vi "encode_test_HOST.vi"() -> ()   [LabVIEW 2014]
uses:
  <vilib>/userdefined/High Color/nirio_resource_hc.ctl
  <vilib>/addons/h5labview2/file/H5Fmode.ctl
  <vilib>/FPGAPlugInAG/PXI-7854R/niLvFpga_Open_PXI-7854R.vi
  <vilib>/rvi/interface/common/dynamic/niFpgaDynamicAddResources.vi
  <vilib>/FPGAPlugInAG/Dynamic/niLvFpga_Run_Dynamic.vi
  <vilib>/Utility/error.llb/Error Cluster From Error Code.vi
  <vilib>/rvi/errors/niLvFpgaAdjustHostInterfaceError.vi
  <vilib>/addons/h5labview2/base/lib_path.vi
  <vilib>/addons/h5labview2/base/H5Equery.vi
  <vilib>/FPGAPlugInAG/Dynamic/niLvFpga_Close_Dynamic.vi
  <vilib>/rvi/interface/nirviOpenFPGA/nirviOpenFPGA.xnode
  FPGA Bitfiles/encodetest,lvpro_FPGATarget_encodetestFPGA_g0rLf42jriM.lvbitx
  <vilib>/rvi/interface/nirviMethod/nirviMethod.xnode
  <vilib>/rvi/interface/nirviReadWriteControl/nirviReadWriteControl.xnode
  <vilib>/addons/h5labview2/base/hid_t.ctl
  <vilib>/addons/h5labview2/dataset/H5Dwrite.llb/H5Dwrite.xnode
  <vilib>/rvi/interface/nirviCloseFPGA/nirviCloseFPGA.xnode
  NiFpgaLv.dll
  <vilib>/rvi/interface/Simulation/niFpgaSimulationCallBeginRW.vi
  <vilib>/rvi/errors/niLvFpgaMergeErrorWithErrorCode.vi
  <vilib>/FPGAPlugInAG/Dynamic/niLvFpga_ReadFifo_Dynamic.vi
  <vilib>/addons/h5labview2/file/H5F.lvlib
  <vilib>/addons/h5labview2/group/H5G.lvlib
  <vilib>/FPGAPlugInAG/Dynamic/niLvFpga_StartFifo_Dynamic.vi
  <vilib>/FPGAPlugInAG/Dynamic/niLvFpga_StopFifo_Dynamic.vi
panel:
  out "loop time":fxp<+,32,32>
  in  "wait (usec)":u32
  in  "Host Update Rate (msec)":dbl=1.0 format="%#_13g"
  in  "Update ADC Clock":bool
  in  "loop timer (usec)":u32=2
  in  "accept_trigs":bool=TRUE
  in  "reset_trigs":bool
  out "config_loaded":bool
  out "fpga_dat_path":path=path "C:/Data/20180605/bead1/discharge/coarse2/turbombar_xyzcool_lessfb_elec3_3000mV41Hz0mVdc_25_fpga.h5"
  out "Nsamp_config":u32=50000
  out "config_trig":bool
  in  "block_hardware_trigs":bool
  out "TRIG0":bool=TRUE
  out "TRIG1":bool=TRUE
  in  "RIO Device":T1="RIO0"
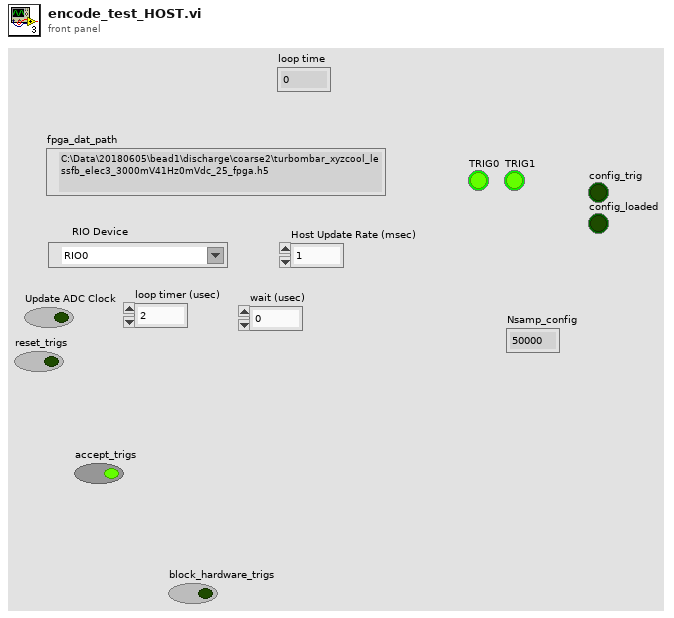
[diagram p1: front panel]
types:
  T1 = typedef "nirio_resource_hc.ctl" = tag
  T2 = enum16{"open", "replace", "create", "open or create", "replace or create", "replace or create with confirmation"}
  T3 = typedef "H5F.lvlib/H5Fmode.ctl" = enum16{"read-only", "read-write", "overwrite", "create new", "open or create"}
  T4 = typedef "hid_t.ctl" = i32
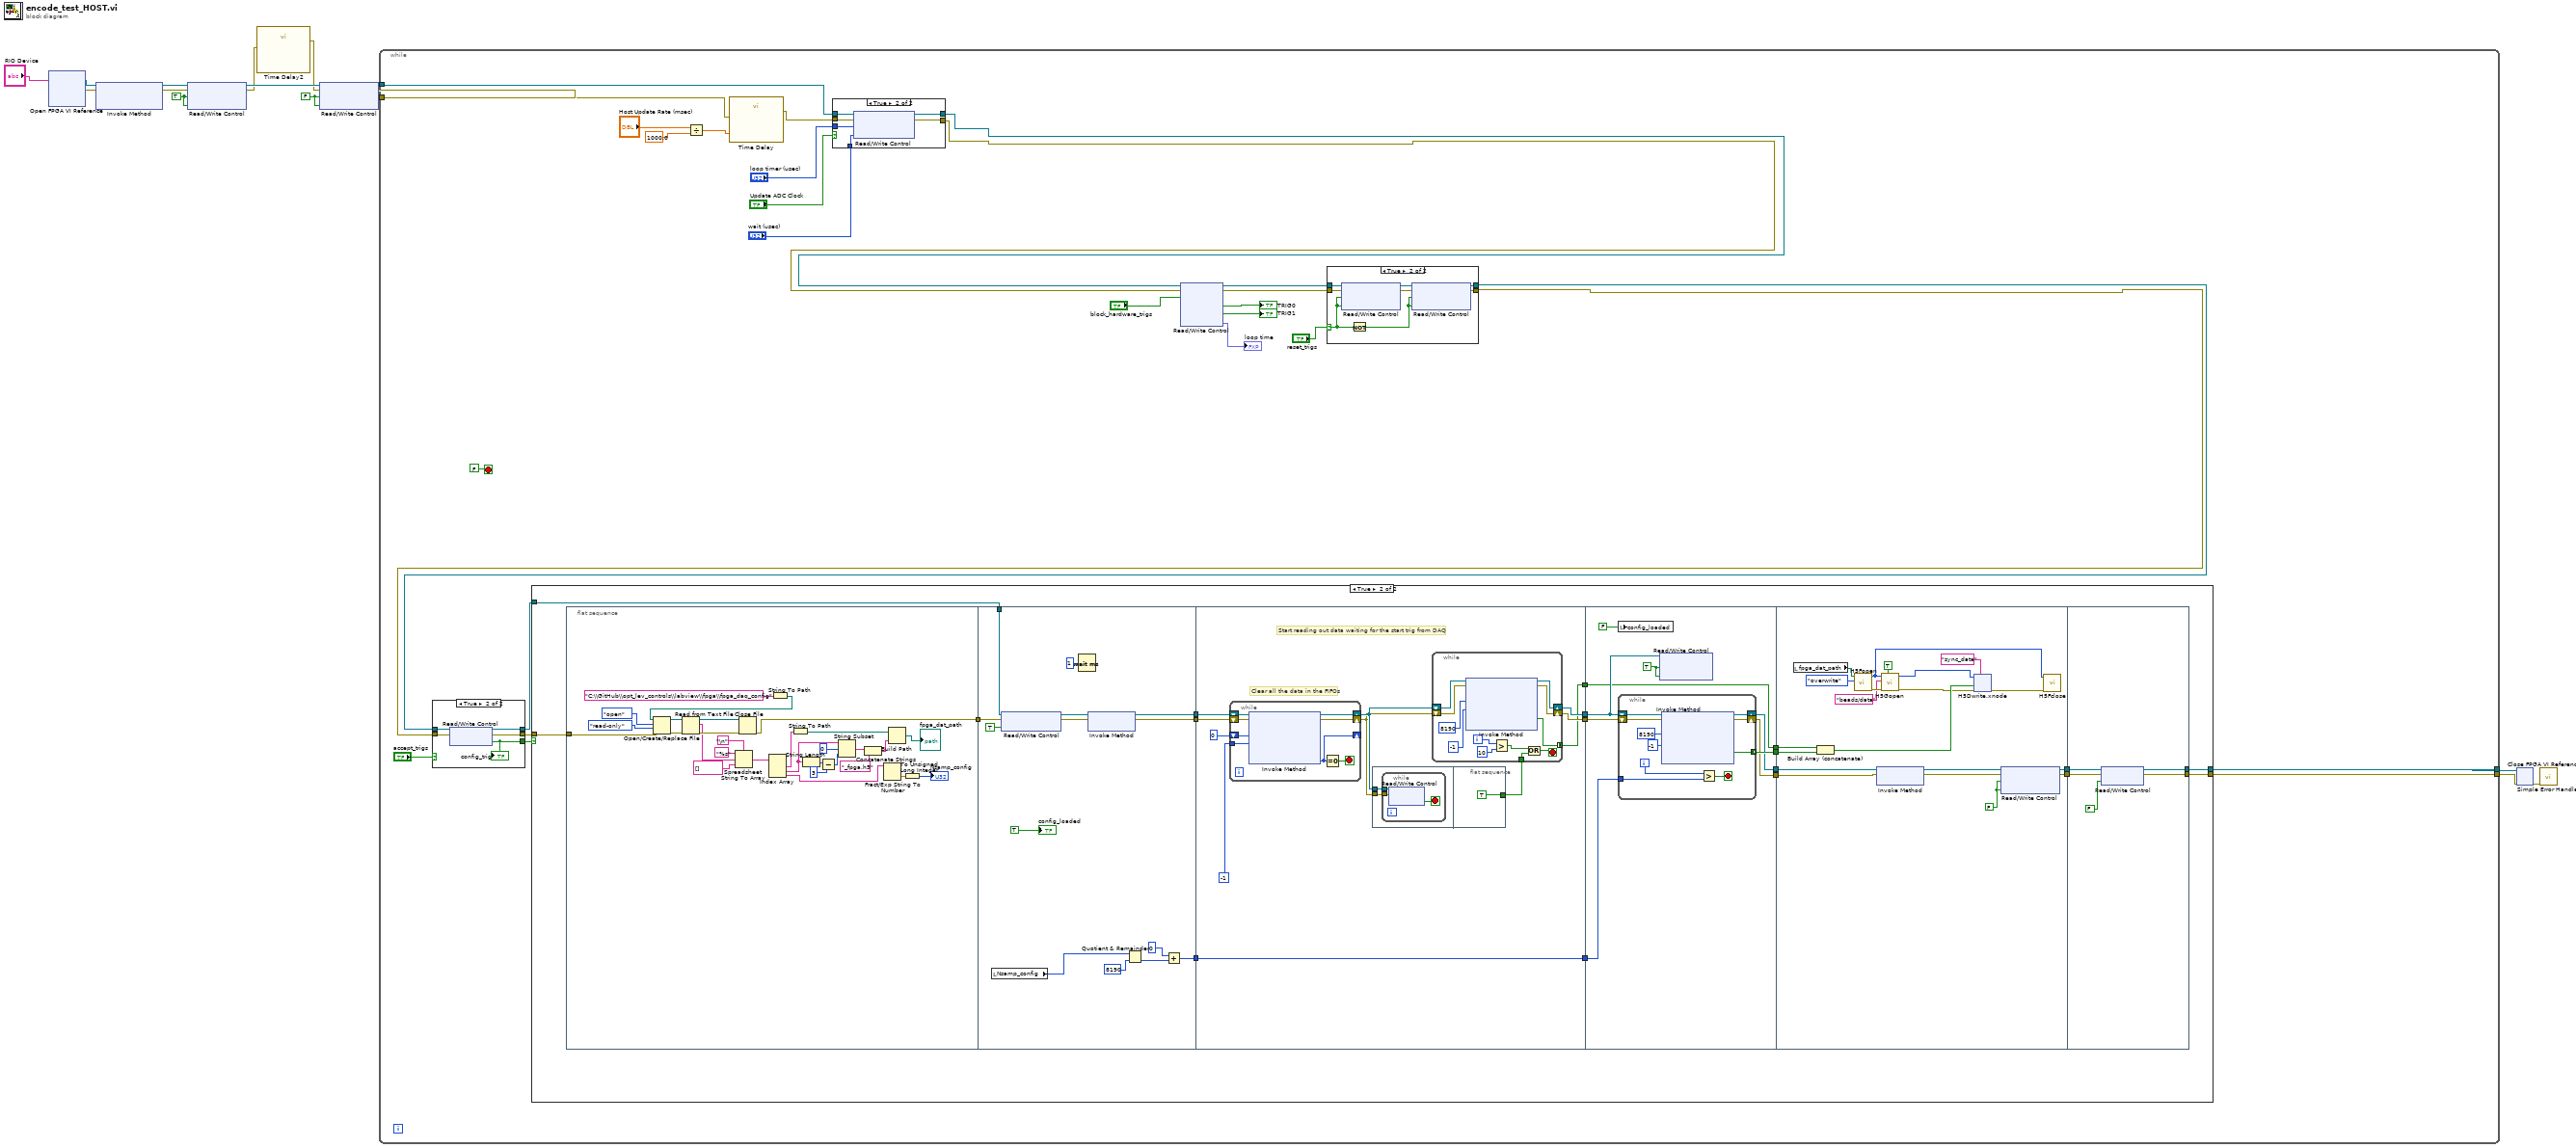
[diagram p0: block diagram]
diagram:
  w5 = FALSE ("manual_trig")
  w3 = TRUE ("reset_trig")
  n1 = xnode "Open FPGA VI Reference"("resource name"="RIO Device") -> ("FPGA VI Reference Out"=w11:refnum<k20>, "error out"=w10:errorcluster)  [unwired: 1 in]
  n2 = xnode "Invoke Method"("FPGA VI Reference In"=w11, "error in"=w10) -> ("FPGA VI Reference Out"=w9:refnum<k20>, "error out"=w8:errorcluster)  [unwired: 1 in]
  n3 = xnode "Read/Write Control"("FPGA VI Reference In"=w9, "error in"=w8, "reset_data_trig"=w3, "reset_config_trig"=w3) -> ("FPGA VI Reference Out"=w4:refnum<k20>, "error out"=w2:errorcluster)
  n4 = call "Time Delay2"("error in (no error)"=w2) -> ("error out"=w1:errorcluster)  [unwired: 10 in]
  n5 = xnode "Read/Write Control"("FPGA VI Reference In"=w4, "error in"=w1, "reset_data_trig"=w5, "reset_config_trig"=w5) -> ("FPGA VI Reference Out"=w7:refnum<k20>, "error out"=w6:errorcluster)
  n6 = while {
    tunnel: w6 -> [w41]
    tunnel: w7 -> [w39]
    tunnel: [w23] -> w14
    tunnel: [w22] -> w13
    stop <- FALSE stop-if-true
    n7 = Divide(x="Host Update Rate (msec)", y=1000.0) -> (x/y=w42:dbl)
    n8 = call "Time Delay"("error in (no error)"=w41, "Delay Time (s)"=w42) -> ("error out"=w38:errorcluster)  [unwired: 9 in]
    n9 = case shown="True" "Update ADC Clock" {
      tunnel: w39 -> [w224 w230]
      tunnel: w38 -> [w223 w229]
      tunnel: [w224 w228] -> w19
      tunnel: [w223 w227] -> w18
      tunnel: "loop timer (usec)" -> [_ w226]
      tunnel: "wait (usec)" -> [_ w225]
      frame False {
      }
      frame True {
        n10 = xnode "Read/Write Control"("FPGA VI Reference In"=w230, "error in"=w229, "loop timer (usec)"=w226, "wait (usec)"=w225) -> ("FPGA VI Reference Out"=w228:refnum<k20>, "error out"=w227:errorcluster)
      }
    }
    n11 = xnode "Read/Write Control"("FPGA VI Reference In"=w19, "error in"=w18, "block_trigs"="block_hardware_trigs") -> ("FPGA VI Reference Out"=w33:refnum<k20>, "error out"=w32:errorcluster, "TRIG0"=→"TRIG0":bool, "TRIG1"=→"TRIG1":bool, "loop time"=→"loop time":fxp<+,32,32>)
    n12 = case shown="True" "reset_trigs" {
      selector: "reset_trigs" -> [_ w216]
      tunnel: w33 -> [w214 w222]
      tunnel: w32 -> [w213 w221]
      tunnel: [w214 w218] -> w21
      tunnel: [w213 w217] -> w20
      frame False {
      }
      frame True {
        n13 = xnode "Read/Write Control"("FPGA VI Reference In"=w222, "error in"=w221, "reset_data_trig"=w216, "reset_config_trig"=w216) -> ("FPGA VI Reference Out"=w220:refnum<k20>, "error out"=w219:errorcluster)
        n14 = Not(x=w216) -> (.not. x?=w215:bool)
        n15 = xnode "Read/Write Control"("FPGA VI Reference In"=w220, "error in"=w219, "reset_data_trig"=w215, "reset_config_trig"=w215) -> ("FPGA VI Reference Out"=w218:refnum<k20>, "error out"=w217:errorcluster)
      }
    }
    n16 = case shown="True" "accept_trigs" {
      selector: "accept_trigs" -> [w45 _]
      tunnel: [w45 w50] -> w29
      tunnel: w20 -> [w43 w49]
      tunnel: w21 -> [w44 w48]
      tunnel: [w44 w47] -> w28
      tunnel: [w43 w46] -> w27
      frame False {
      }
      frame True {
        n17 = xnode "Read/Write Control"("FPGA VI Reference In"=w48, "error in"=w49) -> ("FPGA VI Reference Out"=w47:refnum<k20>, "error out"=w46:errorcluster, "config_trig"=w50:bool)
        "config_trig" <- w50
      }
    }
    n18 = case shown="True" w29 {
      tunnel: w28 -> [w52 w69]
      tunnel: [w52 w58] -> w23
      tunnel: [w51 w57] -> w22
      tunnel: w27 -> [w51 w54]
      frame False {
      }
      frame True {
        n19 = flat-sequence {
          tunnel: [w91] -> w70
          tunnel: w54 -> [w71]
          tunnel: w70 -> [w105]
          tunnel: w69 -> [w106]
          tunnel: [w103] -> w68
          tunnel: [w104] -> w64
          tunnel: [w100] -> w53
          tunnel: w68 -> [w116]
          tunnel: [w120] -> w67
          tunnel: [w119] -> w66
          tunnel: [w118] -> w65
          tunnel: w64 -> [w118]
          tunnel: [w117] -> w62
          tunnel: w53 -> [w115]
          tunnel: w67 -> [w157]
          tunnel: w66 -> [w159]
          tunnel: w65 -> [w158]
          tunnel: [w156] -> w63
          tunnel: w62 -> [w156]
          tunnel: [w155] -> w61
          tunnel: [w154] -> w60
          tunnel: [w153] -> w59
          tunnel: w63 -> [w179]
          tunnel: w61 -> [w178]
          tunnel: w60 -> [w176]
          tunnel: w59 -> [w175]
          tunnel: [w174] -> w56
          tunnel: [w173] -> w55
          tunnel: [w208] -> w57
          tunnel: [w209] -> w58
          tunnel: w56 -> [w211]
          tunnel: w55 -> [w210]
          frame #0 {
            n20 = String To Path(string="C:\\GitHub\\opt_lev_controls\\labview\\fpga\\fpga_daq_config") -> (path=w98:path)
            n21 = Open/Create/Replace File(file path (use dialog)=w98, error in=w71, operation (0:open)=T2."open", access (0:read/write)=enum16{"read/write", "read-only", "write-only"}."read-only") -> (refnum out=w95:refnum<file>, error out=w94:errorcluster)  [unwired: 2 in, 1 out]
            n22 = Read from Text File(file (use dialog)=w95, error in=w94) -> (refnum out=w93:refnum<file>, text=w90:string, error out=w92:errorcluster)  [unwired: 2 in, 1 out]
            n23 = Spreadsheet String To Array(delimiter (Tab)="\n", format string="%s", spreadsheet string=w90, array type (2D Dbl)=string[] [] ("array of strings")) -> (array=w86:string[])
            n24 = Close File(refnum=w93, error in=w92) -> (error out=w91:errorcluster)  [unwired: 1 out]
            n25 = Index Array(array=w86) -> (element #1=w85:string, element #2=w82:string, element #3=w74:string)  [unwired: 3 in]
            n26 = String To Path(string=w85) -> (path=w84:path)
            n27 = String Length(string=w82) -> (length=w81:i32)
            n28 = Subtract(x=w81, y=3) -> (x-y=w79:i32)
            n29 = String Subset(string=w82, offset (0)=0, length (rest)=w79) -> (substring=w78:string)
            n30 = Concatenate Strings(w78, "_fpga.h5" ("string")) -> (w76:string)
            n31 = Fract/Exp String To Number(string=w74) -> (number=w73:dbl)  [unwired: 3 in, 1 out]
            n32 = Build Path(base path=w84, name or relative path=w76) -> (appended path=→"fpga_dat_path":path)
            n33 = To Unsigned Long Integer(number=w73) -> (unsigned 32bit integer=→"Nsamp_config":u32)
          }
          frame #1 {
            n34 = local read "Nsamp_config"() -> (w101:u32)
            n35 = xnode "Read/Write Control"("FPGA VI Reference In"=w106, "error in"=w105, "reset_config_trig"=TRUE) -> ("FPGA VI Reference Out"=w107:refnum<k20>, "error out"=w108:errorcluster)
            n36 = Wait (ms)(milliseconds to wait=u32 1) -> ()  [unwired: 1 out]
            n37 = xnode "Invoke Method"("FPGA VI Reference In"=w107, "error in"=w108) -> ("FPGA VI Reference Out"=w103:refnum<k20>, "error out"=w100:errorcluster)
            n38 = Quotient & Remainder(x=w101, y=u32 8190) -> (floor(x/y)=w111:u32)  [unwired: 1 out]
            n39 = Add(x=u32 0 ("Extra Samps"), y=w111) -> (x+y=w104:u32)
            "config_loaded" <- TRUE
          }
          frame #2 {
            # "Start reading out data waiting for the start trig from DAQ"
            # "Clear all the data in the FIFOs"
            n40 = while {
              tunnel: -1 -> [w145]
              shift-right: [w147] -> w122
              shift-left: w116 -> [w150]
              shift-right: [w146] -> w121
              shift-left: w115 -> [w149]
              shift-right: [w144] -> _
              shift-left: u32 0 ("Elements Remaining") -> [w148]
              stop <- w143 stop-if-true
              n41 = xnode "Invoke Method"("FPGA VI Reference In"=w150, "error in"=w149, "Number of Elements"=w148, "Timeout (ms)"=w145) -> ("FPGA VI Reference Out"=w147:refnum<k20>, "error out"=w146:errorcluster, "Elements Remaining"=w144:u32)  [unwired: 1 out]
              n42 = Equal To 0?(x=w144) -> (x = 0?=w143:bool)
            }
            n43 = flat-sequence {
              tunnel: w122 -> [w126]
              tunnel: w121 -> [w125]
              tunnel: [TRUE] -> w114
              frame #0 {
                n44 = while {
                  tunnel: w126 -> [w129]
                  tunnel: w125 -> [w128]
                  stop <- w127 stop-if-true
                  n45 = xnode "Read/Write Control"("FPGA VI Reference In"=w129, "error in"=w128) -> ("data_trig"=w127:bool)  [unwired: 2 out]
                }
              }
              frame #1 {
              }
            }
            n46 = while {
              tunnel: [w138] -> w117 mode=concatenating
              shift-right: [w140] -> w120
              shift-left: w122 -> [w142]
              shift-right: [w139] -> w119
              shift-left: w121 -> [w141]
              tunnel: w114 -> [w133]
              i -> [w136]
              stop <- w132 stop-if-true
              n47 = xnode "Invoke Method"("FPGA VI Reference In"=w142, "error in"=w141, "Number of Elements"=u32 8190, "Timeout (ms)"=-1) -> ("FPGA VI Reference Out"=w140:refnum<k20>, "error out"=w139:errorcluster, "Data"=w138:bool[])  [unwired: 1 out]
              n48 = Greater?(x=w136, y=10) -> (0:w134:bool)
              n49 = Or(x=w134, y=w133) -> (x .or. y?=w132:bool)
            }
          }
          frame #3 {
            w152 = TRUE
            n50 = local write "config_loaded"(FALSE) -> ()
            n51 = while {
              shift-right: [w165] -> w154
              shift-left: w157 -> [w169]
              shift-right: [w164] -> w153
              shift-left: w159 -> [w168]
              tunnel: w158 -> [w161]
              tunnel: [w160] -> w155 mode=concatenating
              i -> [w163]
              stop <- w162 stop-if-true
              n52 = xnode "Invoke Method"("FPGA VI Reference In"=w169, "error in"=w168, "Number of Elements"=u32 8190, "Timeout (ms)"=-1) -> ("FPGA VI Reference Out"=w165:refnum<k20>, "error out"=w164:errorcluster, "Data"=w160:bool[])  [unwired: 1 out]
              n53 = Greater?(x=w163, y=w161) -> (0:w162:bool)
            }
            n54 = xnode "Read/Write Control"("FPGA VI Reference In"=w157, "reset_data_trig"=w152, "block_trigs"=w152) -> ()  [unwired: 1 in, 2 out]
          }
          frame #4 {
            w187 = FALSE
            n55 = local read "fpga_dat_path"() -> (w182:path)
            n56 = Build Array (concatenate)(w179, w178) -> (w177:bool[])
            n57 = call <vilib>:"H5Fopen.vi"("mode (read-only)"=H5Fmode."overwrite", "path"=w182) -> ("error out"=w186:errorcluster, "ref out"=w180:T4)  [unwired: 8 in]
            n58 = xnode "Invoke Method"("FPGA VI Reference In"=w176, "error in"=w175) -> ("FPGA VI Reference Out"=w188:refnum<k20>, "error out"=w172:errorcluster)
            n59 = call <vilib>:"H5Gopen.vi"("create? (F)"=TRUE, "error in (no error)"=w186, "name"="beads/data", "ref in"=w180) -> ("error out"=w170:errorcluster, "group out"=w181:T4)  [unwired: 6 in]
            n60 = xnode "H5Dwrite.xnode"("dataset name"="sync_data", "error in (no error)"=w170, "data"=w177, "ref in"=w181) -> ("error out"=w171:errorcluster)  [unwired: 3 in, 2 out]
            n61 = xnode "Read/Write Control"("FPGA VI Reference In"=w188, "error in"=w172, "reset_data_trig"=w187, "reset_config_trig"=w187) -> ("FPGA VI Reference Out"=w174:refnum<k20>, "error out"=w173:errorcluster)
            n62 = call <vilib>:"H5Fclose.vi"("error in (no error)"=w171, "ref"=w180) -> ()  [unwired: 9 in, 1 out]
          }
          frame #5 {
            n63 = xnode "Read/Write Control"("FPGA VI Reference In"=w211, "error in"=w210, "block_trigs"=FALSE) -> ("FPGA VI Reference Out"=w209:refnum<k20>, "error out"=w208:errorcluster)
          }
        }
      }
    }
  }
  n64 = xnode "Close FPGA VI Reference"("FPGA VI Reference In"=w14, "error in"=w13) -> ("error out"=w15:errorcluster)
  n65 = call <vilib>:"Simple Error Handler.vi"("error in (no error)"=w15) -> ()  [unwired: 4 in, 5 out]
